vi "GetProtocolList.vi"(4 "password":string="gamma2018", 6 "Username":string="admin", 7 "HTTP_address":string, 8 "error in (no error)":errorcluster, 10 "Value":T2, 11 "Refnum in":T1) -> (0 "error out":errorcluster, 2 "AuthorizationHeader":string, 3 "headers":string)   [LabVIEW 2016]
uses:
  cgi_string.ctl
  <vilib>/httpClient/ClientHandle.ctl
  <vilib>/httpClient/LabVIEWHTTPClient.lvlib
panel:
  in  "Tab Control":enum32{"Server", "Auth"}(tab)
  out "http:":string
  out "body":string
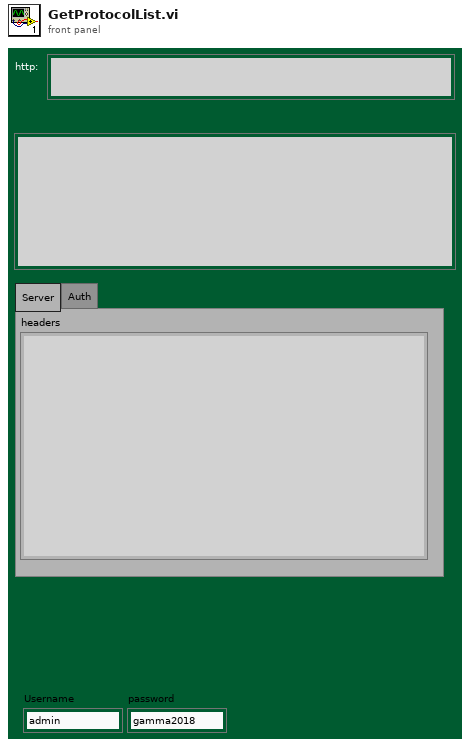
[diagram p1: front panel]
types:
  T1 = typedef "LabVIEWHTTPClient.lvlib/ClientHandle.ctl" = refnum<k1>
  T2 = typedef "cgi_string.ctl" = string
  T3 = cluster{"realm":string, "qop":string, "nounce":string, "opaque":string}
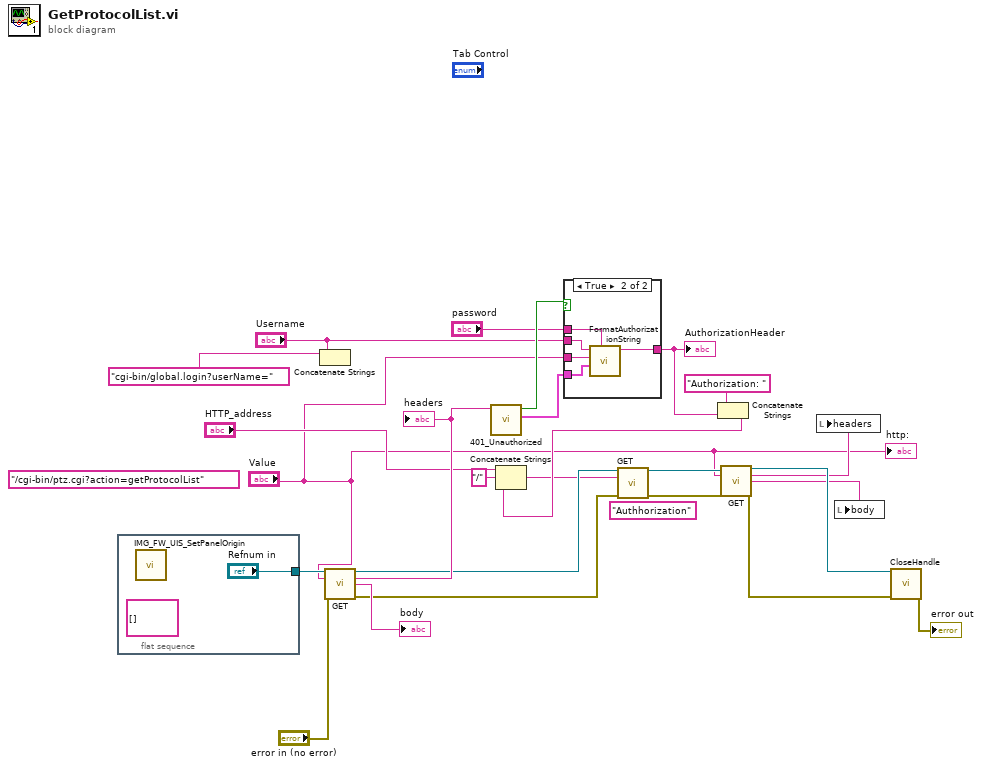
[diagram p0: block diagram]
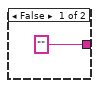
[diagram p2: hidden frame]
diagram:
  (unwired) "Authhorization" ("access id")
  (unwired) T2 "/cgi-bin/ptz.cgi?action=getProtocolList" ("Value")
  n1 = flat-sequence {
    tunnel: ["Refnum in"] -> w22
    frame #0 {
      (unwired) string[][] [] ("Table Control")
      n2 = call "IMG_FW_UIS_SetPanelOrigin.vi"() -> ()  [unwired: 11 in, 1 out]
    }
  }
  n3 = Concatenate Strings("cgi-bin/global.login?userName=", "Username") -> ()  [unwired: 1 out]
  n4 = call <vilib>:"GET.vi"("client handle"=w22, "url"="Value", "error in (no error)"="error in (no error)") -> ("client handle out"=w6:T1, "headers"=w18:string, "body"=→"body":string, "error out"=w15:errorcluster)  [unwired: 9 in]
  "headers" <- w18
  n5 = call "401_Unauthorized.vi"("headers"=w18) -> ("ServerInfo"=w20:T3, "401?"=w21:bool)  [unwired: 8 in, 1 out]
  n6 = case shown="True" w21 {
    tunnel: w20 -> [_ w32]
    tunnel: "Username" -> [_ w31]
    tunnel: "Value" -> [_ w29]
    tunnel: "password" -> [_ w30]
    tunnel: ["" w28] -> w9
    frame False {
    }
    frame True {
      n7 = call "FormatAuthorizationString.vi"("password"=w30, "ServerInfo"=w32, "String in"=w29, "Username"=w31) -> ("String out"=w28:string)  [unwired: 7 in]
    }
  }
  "AuthorizationHeader" <- w9
  n8 = Concatenate Strings("Authorization: " ("string"), w9) -> (w4:string)
  n9 = Concatenate Strings("HTTP_address", "/" ("string"), w4) -> (w3:string)
  n10 = call <vilib>:"GET.vi"("client handle"=w6, "url"=w3, "error in (no error)"=w15) -> ("client handle out"=w8:T1, "error out"=w7:errorcluster)  [unwired: 9 in, 2 out]
  n11 = call <vilib>:"GET.vi"("client handle"=w8, "url"="Value", "error in (no error)"=w7) -> ("client handle out"=w16:T1, "headers"=w12:string, "body"=w13:string, "error out"=w14:errorcluster)  [unwired: 9 in]
  n12 = local write "headers"(w12) -> ()
  n13 = local write "body"(w13) -> ()
  n14 = call <vilib>:"CloseHandle.vi"("client handle"=w16, "error in (no error)"=w14) -> ("error out"=→"error out":errorcluster)  [unwired: 13 in]
  "http:" <- "Value"
